vi "Cycle.vi"(8 "error in":errorcluster, 11 "Teir":T1) -> ()   [LabVIEW 2014, in "Elevator System.lvlib"]
uses:
  Elevator System.lvlib
  Typedef/TeirNumber.ctl
  Typedef/MessageType.ctl
  Typedef/Commands.ctl
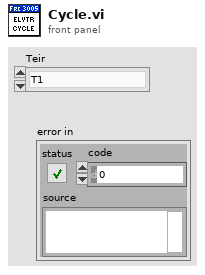
[diagram p1: front panel]
types:
  T1 = typedef "Elevator System.lvlib/TeirNumber.ctl" = enum16{"T1", "T2", "T3", "T4", "T5", "T6"}
  T2 = typedef "Elevator System.lvlib/Commands.ctl" = enum16{"Home", "Stack", "Pickup", "Score", "Cycle", "Stop", "Manual Open", "Manual Close", "Manual Up", "Manual Down", "Gripper RC", "Gripper Cycle", "Wait On Gripper", "Wait On Elevator"}
  T3 = typedef "Elevator System.lvlib/MessageType.ctl" = cluster{"Name":T2, "Data":variant}
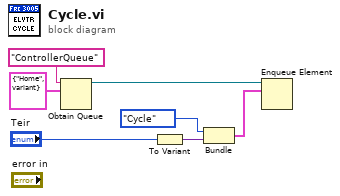
[diagram p0: block diagram]
diagram:
  n1 = Obtain Queue(name (unnamed)="ControllerQueue", element data type=T3 {"Name"=enum."Home", "Data"=variant} ("Message")) -> (queue out=w7:refnum<queue>)  [unwired: 3 in, 2 out]
  n2 = To Variant(anything="Teir") -> (Variant=w5:variant)
  n3 = Bundle("Name"=Commands."Cycle", "Variant"=w5) -> (w3:cluster{"Name":T2, "Variant":variant})  [unwired: 1 in]
  n4 = Enqueue Element(queue=w7, element=w3) -> ()  [unwired: 2 in, 3 out]
